vi "CSDB_Common.get id.vi"(0 "connection reference":T1, 2 "Class/Attribute/Instance Name":string, 3 "Table":enum16{"Classes", "Attributes", "Instances"}(ring), 5 "error in (no error)":errorcluster, 10 "check existing ?":bool) -> (14 "connection reference out":T1, 16 "ID string":string, 17 "ID":i32, 19 "error out":errorcluster)   [LabVIEW 2014, in "CSDB_Common.lvlib"]
doc: "Returns the ID in the CSDatabase of a Class/Attribute or Instance. \n<B>ID = -1</B> - entry doesnt exist. \n<B>ID = 0</B> - error in = True\n!!! If <B>check existing?</B> is false but the entry doesnt exist \nthe function may return senseless values !!!\n(If <B>error in</B> is false any errors inside are ignored and <B>error out</B> is false )"
uses:
  CSDB_Common.lvlib
  <vilib>/addons/database/Connection.llb/Conn ObjectReference.ctl
  <vilib>/addons/database/NI_Database_API.lvlib
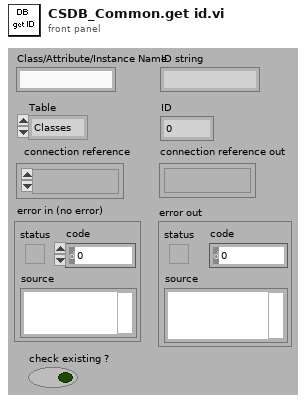
[diagram p1: front panel]
types:
  T1 = typedef "NI_Database_API.lvlib/Conn ObjectReference.ctl" = refnum<k1>
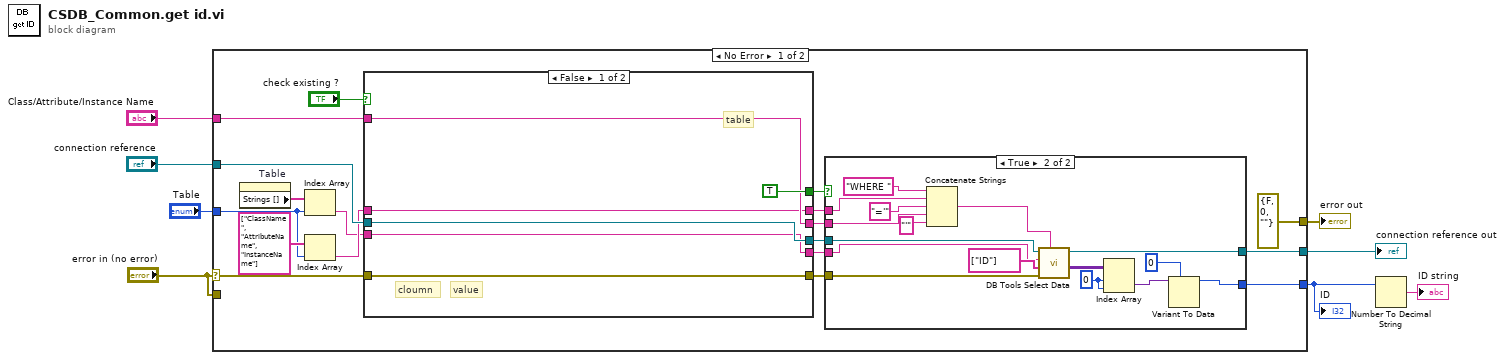
[diagram p0: block diagram]
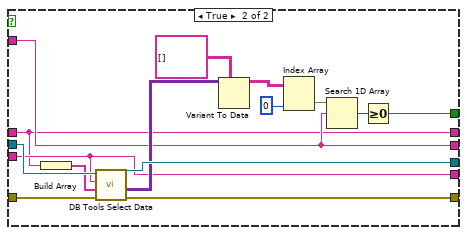
[diagram p2: hidden frame]
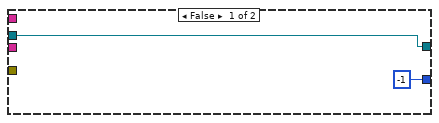
[diagram p3: hidden frame]
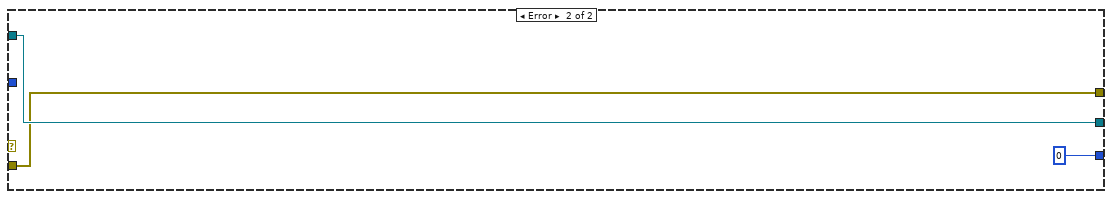
[diagram p4: hidden frame]
diagram:
  n1 = case shown="No Error" "error in (no error)" {
    selector: "error in (no error)" -> [w21 _]
    tunnel: "connection reference" -> [w19 w68]
    tunnel: "error in (no error)" -> [_ w66]
    tunnel: "Table" -> [w24 _]
    tunnel: "Class/Attribute/Instance Name" -> [w16 _]
    tunnel: [w23 w68] -> w5
    tunnel: [w22 0] -> w3
    tunnel: [errorcluster {"status"=FALSE, "code"=0, "source"=""} ("error in (no error)") w66] -> w1
    frame No Error {
      n2 = property on="Table" class="Enum (strict)"() -> ("Strings []"=w26:string[])  [unwired: 2 in, 2 out]
      n3 = Index Array(array=w26, index=w24) -> (element=w14:string)
      n4 = Index Array(array=string[] ["ClassName", "AttributeName", "InstanceName"], index=w24) -> (element=w17:string)
      n5 = case shown="False" "check existing ?" {
        tunnel: w21 -> [w30 w47]
        tunnel: [w30 w46] -> w20
        tunnel: w19 -> [w31 w45]
        tunnel: [w31 w44] -> w18
        tunnel: w17 -> [w27 w33]
        tunnel: w16 -> [w28 w34]
        tunnel: [TRUE w43] -> w15
        tunnel: w14 -> [w29 w35]
        tunnel: [w29 w35] -> w13
        tunnel: [w28 w34] -> w12
        tunnel: [w27 w33] -> w11
        frame False {
          # "table"
          # "value"
          # "cloumn"
        }
        frame True {
          n6 = Build Array(w33) -> (w42:string[])
          n7 = call <vilib>:"DB Tools Select Data.vi"("error in (no error)"=w47, "columns"=w42, "table"=w35, "connection reference"=w45) -> ("error out"=w46:errorcluster, "data"=w41:variant[][], "connection reference out"=w44:T1)  [unwired: 2 in]
          n8 = Variant To Data(type=string[][] [], Variant=w41) -> (data=w39:string[][])  [unwired: 1 in, 1 out]
          n9 = Index Array(array=w39, index (col)=0 ("disabled index (col)")) -> (element=w37:string[])  [unwired: 1 in]
          n10 = Search 1D Array(1D array=w37, element=w34) -> (index of element=w36:i32)  [unwired: 1 in]
          n11 = Greater Or Equal To 0?(x=w36) -> (x >= 0?=w43:bool)
        }
      }
      n12 = case shown="True" w15 {
        tunnel: [w49 w61] -> w23
        tunnel: [-1 w56] -> w22
        tunnel: w20 -> [_ w54]
        tunnel: w18 -> [w49 w53]
        tunnel: w13 -> [_ w52]
        tunnel: w11 -> [_ w51]
        tunnel: w12 -> [_ w50]
        frame False {
        }
        frame True {
          w59 = 0 ("index (row)")
          n13 = Concatenate Strings("WHERE " ("optional clause"), w51, "='" ("string"), w50, "'" ("string")) -> (w62:string)
          n14 = call <vilib>:"DB Tools Select Data.vi"("condition"=w62, "error in (no error)"=w54, "columns"=string[] ["ID"], "table"=w52, "connection reference"=w53) -> ("data"=w60:variant[][], "connection reference out"=w61:T1)  [unwired: 1 in, 1 out]
          n15 = Index Array(array=w60, index (row)=w59, index (col)=w59) -> (element=w58:variant)
          n16 = Variant To Data(type=0, Variant=w58) -> (data=w56:i32)  [unwired: 1 in, 1 out]
        }
      }
    }
    frame Error {
    }
  }
  "connection reference out" <- w5
  "ID" <- w3
  "error out" <- w1
  n17 = Number To Decimal String(number=w3) -> (decimal integer string=→"ID string":string)  [unwired: 1 in]
